vi "edge_detect.vi"() -> ()   [LabVIEW 2020]
uses:
  <vilib>/userDefined/High Color/IMAQdx.ctl
  <vilib>/vision/Image Controls.llb/IMAQ Image.ctl
  <vilib>/Analysis/baseanly.llb/Real A x B.vi
  <vilib>/Analysis/Matrix/Numeric/Conversions/Array To Matrix - RA.vi
  <vilib>/Analysis/Matrix/Numeric/Conversions/Matrix To Array - RM.vi
  <vilib>/vision/driver/NI_Vision_Acquisition_Software.lvlib
  <vilib>/Analysis/Matrix/NI_Matrix.lvlib
  <vilib>/Analysis/NI_AALBase.lvlib
panel:
  in  "stop":bool
  out "output cluster 2":cluster{dbl, dbl}
  out "output cluster":cluster{dbl, dbl}
  out "Image Out":T1
  in  "Cam Setting":T2
  out "Image":T1(plugin-control)
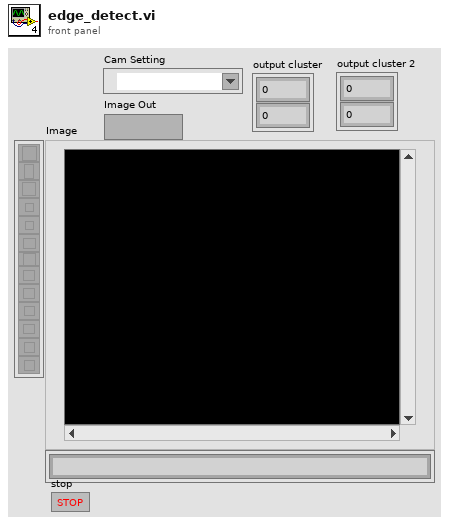
[diagram p1: front panel]
types:
  T1 = typedef "IMAQ Image.ctl" = refnum<image>
  T2 = typedef "IMAQdx.ctl" = refnum<k21>
  T3 = typedef "Image Type" = u32
  T4 = cluster{"Global Rectangle":i32[], "Contours":cluster{"Contour Type":u32, "ROI Type":u32, "Points":i32[]}[]}
  T5 = cluster{"Point1 (Pixels)":cluster{"X":sgl, "Y":sgl}, "Point2 (Pixels)":cluster{"X":sgl, "Y":sgl}, "Point1 (Real-World)":cluster{"X":sgl, "Y":sgl}, "Point2 (Real-World)":cluster{"X":sgl, "Y":sgl}, "Angle (Pixel)":dbl, "Angle (Real-World)":dbl, "Score":dbl, "Straightness":dbl, "Average SNR (db)":dbl, "Calibration Valid":bool}[]
  T6 = cluster{"Point1 (Pixels)":cluster{"X":sgl, "Y":sgl}, "Point2 (Pixels)":cluster{"X":sgl, "Y":sgl}, "Point1 (Real-World)":cluster{"X":sgl, "Y":sgl}, "Point2 (Real-World)":cluster{"X":sgl, "Y":sgl}, "Angle (Pixel)":dbl, "Angle (Real-World)":dbl, "Score":dbl, "Straightness":dbl, "Average SNR (db)":dbl, "Calibration Valid":bool}
  T7 = typedef "NI_Matrix.lvlib/RealMatrix.ctl" = dbl[][]
  T8 = cluster{"Real 2D Array[0]":dbl, "Real 2D Array[1]":dbl, "Real 2D Array[2]":dbl, "Real 2D Array[3]":dbl, "Real 2D Array[4]":dbl, "Real 2D Array[5]":dbl, "Real 2D Array[6]":dbl, "Real 2D Array[7]":dbl, "Real 2D Array[8]":dbl}
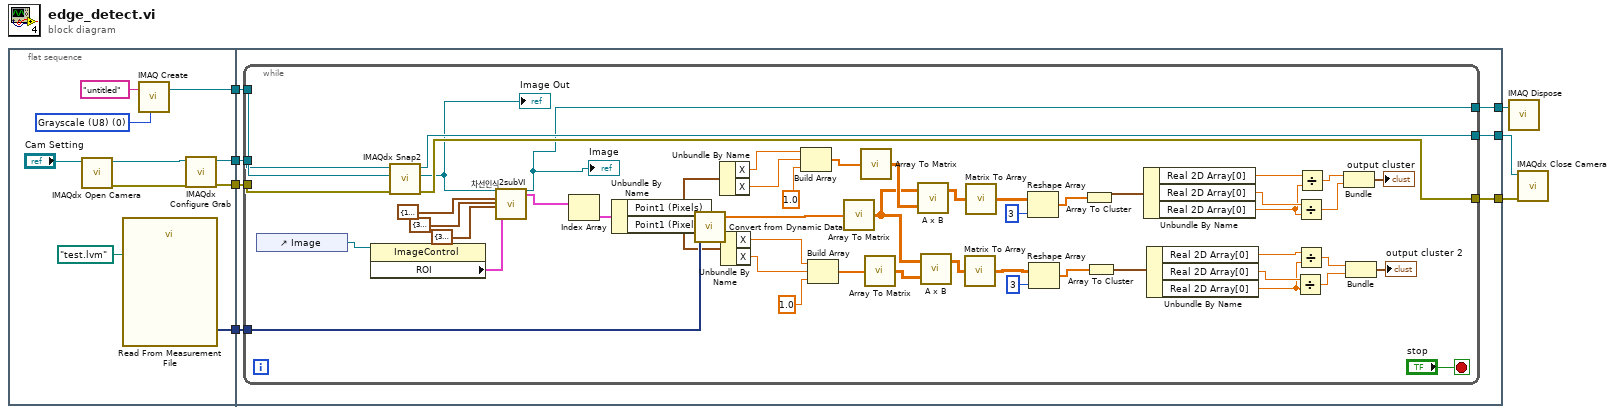
[diagram p0: block diagram]
diagram:
  n1 = flat-sequence {
    tunnel: [w11] -> w7
    tunnel: [w10] -> w6
    tunnel: [w9] -> w5
    tunnel: [w8] -> w4
    tunnel: w7 -> [w23]
    tunnel: w6 -> [w21]
    tunnel: w5 -> [w22]
    tunnel: w4 -> [w24]
    tunnel: [w20] -> w3
    tunnel: [w19] -> w2
    tunnel: [w18] -> w1
    frame #0 {
      w12 = T3 0 items=["Grayscale (U8)", "Grayscale (I16)", "Grayscale (SGL)", "Complex (CSG)", "RGB (U32)", "HSL (U32)", "RGB (U64)", "Grayscale (U16)"] ("Image Type")
      n2 = call <vilib>:"IMAQdx Open Camera.vi"("Session In"="Cam Setting") -> ("error out"=w15:errorcluster, "Session Out"=w16:T2)  [unwired: 9 in]
      n3 = call "Read From Measurement File"("Filename"=path "test.lvm") -> ("Signals"=w8:dynamicdata)  [unwired: 5 in, 5 out]
      n4 = call "IMAQ Create"("Image Name"="untitled", "Image Type"=w12) -> ("New Image"=w11:T1)  [unwired: 3 in, 1 out]
      n5 = call <vilib>:"IMAQdx Configure Grab.vi"("error in"=w15, "Session In"=w16) -> ("error out"=w9:errorcluster, "Session Out"=w10:T2)  [unwired: 8 in]
    }
    frame #1 {
      n6 = while {
        tunnel: w24 -> [w75]
        tunnel: w23 -> [w74]
        tunnel: w22 -> [w73]
        tunnel: w21 -> [w72]
        tunnel: [w28] -> w20
        tunnel: [w27] -> w19
        tunnel: [w25] -> w18
        stop <- "stop" stop-if-true
        n7 = control-ref of="Image"() -> (w76:refnum<vi>)
        n8 = property class="ImageControl"(reference=w76) -> ("ROI"=w33:T4)  [unwired: 1 in, 2 out]
        n9 = call <vilib>:"IMAQdx Snap2.vi"("error in"=w73, "Image In"=w74, "Session In"=w72) -> ("error out"=w27:errorcluster, "Image Out"=w26:T1, "Session Out"=w28:T2)  [unwired: 6 in]
        "Image Out" <- w26
        n10 = call "차선인식2subVI.vi"("Image In"=w26, "Red or Hue Range (Color Threshold 1)"=cluster{"Lower value":i32, "Upper value":i32} {"Lower value"=17, "Upper value"=214}, "Green or Sat Range (Color Threshold 1)"=cluster{"Lower value":i32, "Upper value":i32} {"Lower value"=35, "Upper value"=255}, "Blue or Luma or Val or Inten Range (Color Threshold 1)"=cluster{"Lower value":i32, "Upper value":i32} {"Lower value"=38, "Upper value"=178}, "ROI Descriptor (Adv. Straight Edge 1)"=w33) -> ("Image Out"=w25:T1, "Straight Edges (Adv. Straight Edge 1)"=w32:T5)  [unwired: 15 in, 6 out]
        "Image" <- w25
        n11 = Index Array(array=w32) -> (element=w71:T6)  [unwired: 1 in]
        n12 = Unbundle By Name(w71) -> ("Point1 (Pixels)"=w69:cluster{"X":sgl, "Y":sgl}, "Point1 (Pixels)"=w70:cluster{"X":sgl, "Y":sgl})
        n13 = call "Convert from Dynamic Data"("Dynamic Data Type"=w75) -> ("Array"=w60:dbl[])  [unwired: 3 in]
        n14 = Unbundle By Name(w69) -> ("X"=w68:sgl, "X"=w67:sgl)
        n15 = Unbundle By Name(w70) -> ("X"=w66:sgl, "X"=w65:sgl)
        n16 = Build Array(w68, w67, 1.0) -> (w62:dbl[])
        n17 = Build Array(w66, w65, 1.0) -> (w61:dbl[])
        n18 = call-poly <vilib>:"Array To Matrix.vi"("Real 1D Array"=w60) -> ("Real Matrix (Column Vector)"=w57:T7)
        n19 = call-poly <vilib>:"Array To Matrix.vi"("Real 1D Array"=w62) -> ("Real Matrix (Column Vector)"=w59:T7)
        n20 = call-poly <vilib>:"Array To Matrix.vi"("Real 1D Array"=w61) -> ("Real Matrix (Column Vector)"=w58:T7)
        n21 = call-poly <vilib>:"A x B.vi"("B"=w59, "A"=w57) -> ("A x B"=w52:T7)  [unwired: 1 out]
        n22 = call-poly <vilib>:"A x B.vi"("B"=w58, "A"=w57) -> ("A x B"=w50:T7)  [unwired: 1 out]
        n23 = call-poly <vilib>:"Matrix To Array.vi"("Real Matrix"=w50) -> ("Real 2D Array"=w49:dbl[][])
        n24 = call-poly <vilib>:"Matrix To Array.vi"("Real Matrix"=w52) -> ("Real 2D Array"=w51:dbl[][])
        n25 = Reshape Array(w51, 3 ("dimension size")) -> (w53:dbl[])
        n26 = Reshape Array(w49, 3 ("dimension size")) -> (w54:dbl[])
        n27 = Array To Cluster(array=w53) -> (cluster=w48:T8)
        n28 = Array To Cluster(array=w54) -> (cluster=w47:T8)
        n29 = Unbundle By Name(w48) -> ("Real 2D Array[0]"=w46:dbl, "Real 2D Array[0]"=w45:dbl, "Real 2D Array[0]"=w44:dbl)
        n30 = Unbundle By Name(w47) -> ("Real 2D Array[0]"=w43:dbl, "Real 2D Array[0]"=w42:dbl, "Real 2D Array[0]"=w41:dbl)
        n31 = Divide(x=w42, y=w41) -> (x/y=w37:dbl)
        n32 = Divide(x=w45, y=w44) -> (x/y=w39:dbl)
        n33 = Divide(x=w43, y=w41) -> (x/y=w38:dbl)
        n34 = Divide(x=w46, y=w44) -> (x/y=w40:dbl)
        n35 = Bundle(w40, w39) -> (→"output cluster":cluster{dbl, dbl})  [unwired: 1 in]
        n36 = Bundle(w38, w37) -> (→"output cluster 2":cluster{dbl, dbl})  [unwired: 1 in]
      }
    }
  }
  n37 = call "IMAQ Dispose"("Image"=w1) -> ()  [unwired: 5 in, 1 out]
  n38 = call <vilib>:"IMAQdx Close Camera.vi"("error in"=w2, "Session In"=w3) -> ()  [unwired: 9 in, 1 out]
